vi "getpagesize.vi"(8 "error in (no error)":errorcluster) -> (0 "error out":errorcluster, 3 "page size":u32)   [LabVIEW 2013, in "Linux RT IPC.lvlib" / "Shared Memory.lvlib" / "Shared Memory.lvclass"]
doc: "Wrapper VI for Linux function getpagesize()."
uses:
  Shared Memory.lvclass
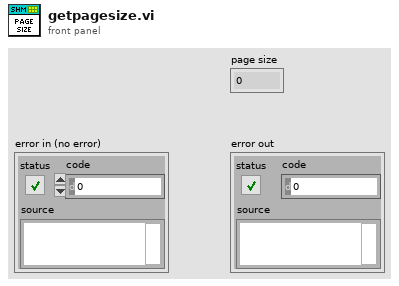
[diagram p1: front panel]
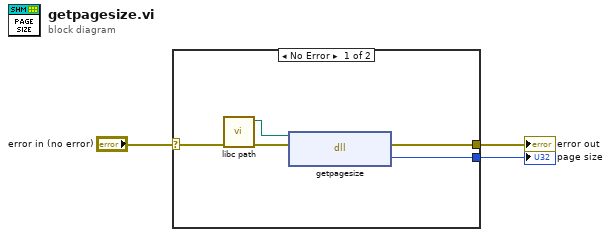
[diagram p0: block diagram]
diagram:
  n1 = case shown="No Error" "error in (no error)" {
    selector: "error in (no error)" -> [w6 w9]
    tunnel: [w8 w9] -> w3
    tunnel: [w7 _] -> w2
    frame No Error {
      n2 = call "libc path.vi"("error in (no error)"=w6) -> ("error out"=w5:errorcluster, "path to libc"=w4:path)  [unwired: 9 in]
      n3 = dll-call lib="?" fn="getpagesize"(path in=w4, error in=w5) -> (error out=w8:errorcluster, "page size"=w7:u32)  [unwired: 1 in, 1 out]
    }
    frame Error {
    }
  }
  "error out" <- w3
  "page size" <- w2
